vi "Do Command.vi"(6 "Timing":T1, 7 "Variables in":refnum<class "Variables.lvclass">, 8 "error in (no error)":errorcluster, 10 "VolatusAPI":refnum<class "VolatusAPI.lvclass">, 11 "Command in":refnum<class "Command.lvclass">) -> (0 "error out":errorcluster, 3 "Command out":refnum<class "Command.lvclass">, 5 "Variables":refnum<class "Variables.lvclass">)   [LabVIEW 2020, in "VolatusSeq.lvlib" / "Command.lvclass"]
uses:
  Command.lvclass
  Command.lvclass/Command.ctl
  Variables/Variables.lvclass
  Timing.ctl
  VolatusSeq.lvlib
  Volatus/VolatusAPI/VolatusAPI.lvclass
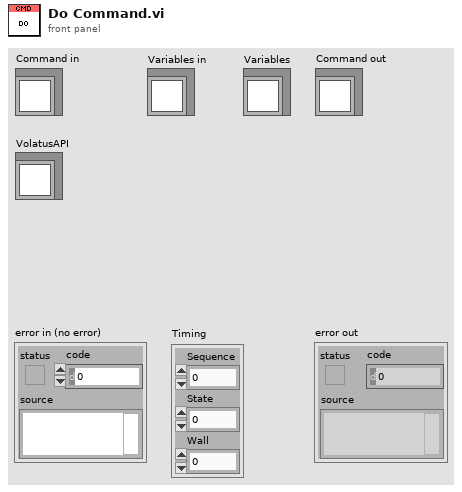
[diagram p1: front panel]
types:
  T1 = typedef "VolatusSeq.lvlib/Timing.ctl" = cluster{"Sequence":dbl, "State":dbl, "Wall":dbl}
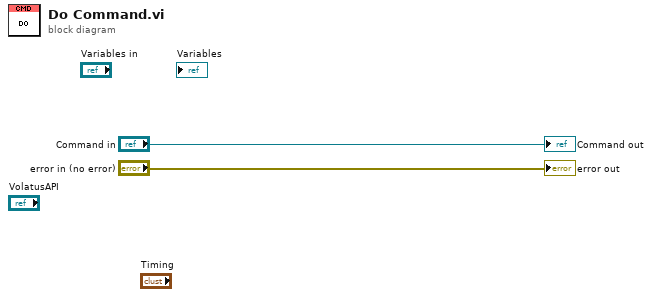
[diagram p0: block diagram]
diagram:
  "error out" <- "error in (no error)"
  "Command out" <- "Command in"
